vi "Status.vi"(0 "Notifier Name":string, 11 "Error In":errorcluster) -> (4 "Notifier Name Dup":string, 6 "Filter Wheel":i32=1 min=1 max=8, 8 "Dichroic":i32=1 min=1 max=5, 10 "Disk Position":i32 min=0 max=2, 13 "Disk On":bool, 15 "Error Out":errorcluster)   [LabVIEW 2020]
uses:
  Spinning Disk Type Defs/SD Notifer Data.ctl
  Spinning Disk Type Defs/SD Actions.ctl
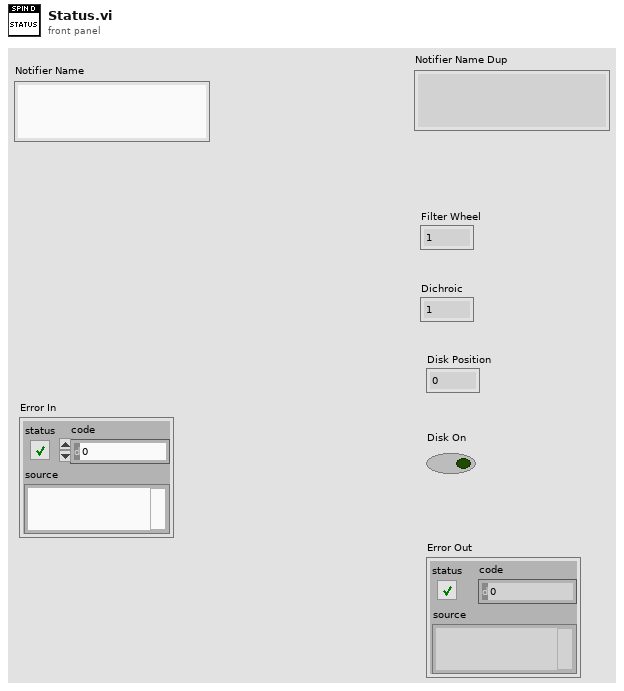
[diagram p1: front panel]
types:
  T1 = typedef "SD Notifer Data.ctl" = cluster{"Actions":T2, "Disk On?":bool, "Dichroic Pos.":i32, "Filter Wheel Pos.":i32, "Disk Pos.":i32, "Recived":bool}
  T2 = typedef "SD Actions.ctl" = enum16{"Status", "Get All Pos.", "Home All", "Set Filter Wheel Pos.", "Set Disk Pos.", "Set Dichroic Pos.", "Disk On", "Disk Off", "Quit"}
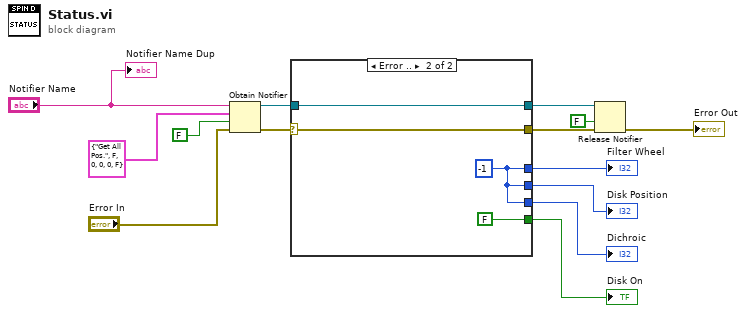
[diagram p0: block diagram]
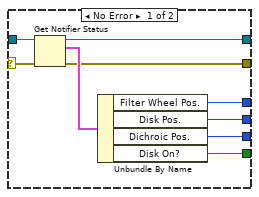
[diagram p2: hidden frame]
diagram:
  n1 = Obtain Notifier(name (unnamed)="Notifier Name", notification data type=T1 {"Actions"=enum."Get All Pos.", "Disk On?"=FALSE, "Dichroic Pos."=0, "Filter Wheel Pos."=0, "Disk Pos."=0, "Recived"=FALSE} ("XLight Notifier Data"), create if not found? (T)=FALSE, error in (no error)="Error In") -> (notifier out=w10:refnum<notifier>, error out=w7:errorcluster)  [unwired: 1 out]
  n2 = case shown="Error .." w7 {
    selector: w7 -> [w16 w26]
    tunnel: w10 -> [w23 w27]
    tunnel: [w22 w27] -> w9
    tunnel: [w20 w25] -> w5
    tunnel: [w19 w25] -> w4
    tunnel: [w18 w25] -> w3
    tunnel: [w17 FALSE ("Disk On?")] -> w2
    tunnel: [w15 w26] -> w6
    frame No Error {
      n3 = Get Notifier Status(notifier=w23, error in (no error)=w16) -> (notifier out=w22:refnum<notifier>, current notification=w21:T1, error out=w15:errorcluster)  [unwired: 2 out]
      n4 = Unbundle By Name(w21) -> ("Filter Wheel Pos."=w20:i32, "Disk Pos."=w19:i32, "Dichroic Pos."=w18:i32, "Disk On?"=w17:bool)
    }
    frame Error {
      w25 = -1 ("Filter Wheel Pos.")
    }
  }
  "Filter Wheel" <- w5
  "Dichroic" <- w3
  "Disk Position" <- w4
  "Disk On" <- w2
  n5 = Release Notifier(notifier=w9, force destroy? (F)=FALSE, error in (no error)=w6) -> (error out=→"Error Out":errorcluster)  [unwired: 2 out]
  "Notifier Name Dup" <- "Notifier Name"
